vi "Transmit Datagram.vi"(5 "transfer id":i32, 7 "transfer group id":i32, 8 "error in (no error)":errorcluster, 9 "transfer data":string, 11 "UDPlog Transceiver in":refnum<class "UDPlog Transceiver.lvclass">) -> (0 "error out":errorcluster, 1 "timed out?":bool, 3 "UDPlog Transceiver out":refnum<class "UDPlog Transceiver.lvclass">)   [LabVIEW 2023, in "UDPlog.lvlib" / "UDPlog Transceiver.lvclass"]
uses:
  UDPlog Transceiver.lvclass
  UDPlog Transceiver.lvclass/UDPlog Transceiver.ctl
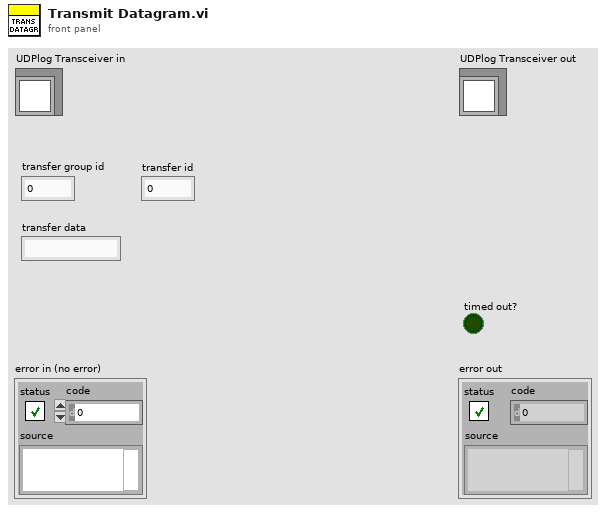
[diagram p1: front panel]
types:
  T1 = typedef "UDPlog.lvlib/UDPlog Transceiver.lvclass/Trasfer Group Parameters.ctl" = cluster{"transfers":T2[], "max size":i32, "timeout":i32}
  T2 = typedef "UDPlog.lvlib/UDPlog Transceiver.lvclass/Transfer Parameters.ctl" = cluster{"group offset":u64, "size":u64, "address":u32, "port":u16}
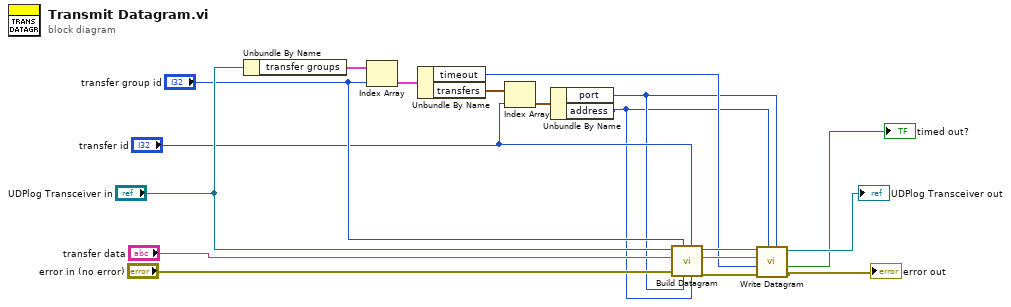
[diagram p0: block diagram]
diagram:
  n1 = Unbundle By Name("UDPlog Transceiver in") -> ("transfer groups"=w15:T1[])
  n2 = Index Array(array=w15, index="transfer group id") -> (element=w16:T1)
  n3 = Unbundle By Name(w16) -> ("timeout"=w4:i32, "transfers"=w18:T2[])
  n4 = Index Array(array=w18, index="transfer id") -> (element=w17:T2)
  n5 = Unbundle By Name(w17) -> ("port"=w3:u16, "address"=w2:u32)
  n6 = call-dynamic "Build Datagram.vi"("destination address"=w2, "transfer id"="transfer id", "destination port"=w3, "transfer group id"="transfer group id", "error in (no error)"="error in (no error)", "transfer data"="transfer data", "UDPlog Transceiver in"="UDPlog Transceiver in") -> ("error out"=w6:errorcluster, "datagram"=w5:string, "UDPlog Transceiver out"=w9:refnum<class "UDPlog Transceiver.lvclass">)  [unwired: 2 in]
  n7 = call "Write Datagram.vi"("destination port"=w3, "destination address"=w2, "error in (no error)"=w6, "timeout ms (25000)"=w4, "data"=w5, "UDPlog Transceiver in"=w9) -> ("error out"=→"error out":errorcluster, "timed out?"=→"timed out?":bool, "UDPlog Transceiver out"=→"UDPlog Transceiver out":refnum<class "UDPlog Transceiver.lvclass">)  [unwired: 3 in]
